vi "Spawn TCP Service.vi"(4 "Stop Module":refnum<user-event>, 6 "Message Queue":refnum<class "Delacor_lib_QMH_Message Queue.lvclass">, 7 "GenNet Protocol":refnum<class "GenNet Protocol.lvclass">, 8 "error in":errorcluster, 9 "Module ID":i32=-1, 11 "Connection ID":refnum<k5>) -> (0 "error out":errorcluster)   [LabVIEW 2022 SP3, in "GenNet-Server.lvlib"]
doc: "Spawns a new TCP/IP service for a networked client. Sets <b>Connection ID</b> reference, <b>Module ID</b>, <b>Caller MsqQ</b> queue reference and <b>Stop Module</b> event reference before running the service VI.\n\n____\nHAMPEL SOFTWARE ENGINEERING v3.8.0 (2023-12-18 14:41)"
uses:
  GenNet-Server.lvlib
  <vilib>/Delacor/Delacor QMH/Libraries/Message Queue_class/Delacor_lib_QMH_Message Queue.lvclass
  Stop Argument--cluster.ctl
  GenNet Protocols/GenNet Protocol.lvclass
  TCP Service.vi
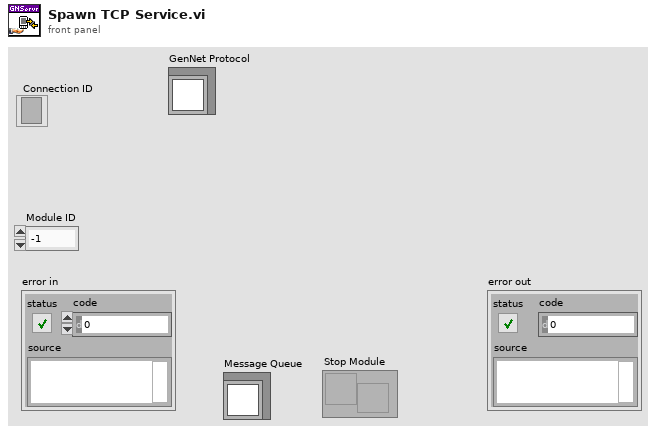
[diagram p1: front panel]
types:
  T1 = enum32{"Invalid", "Standard", "Closed", "Hidden", "Minimized", "Maximized"}
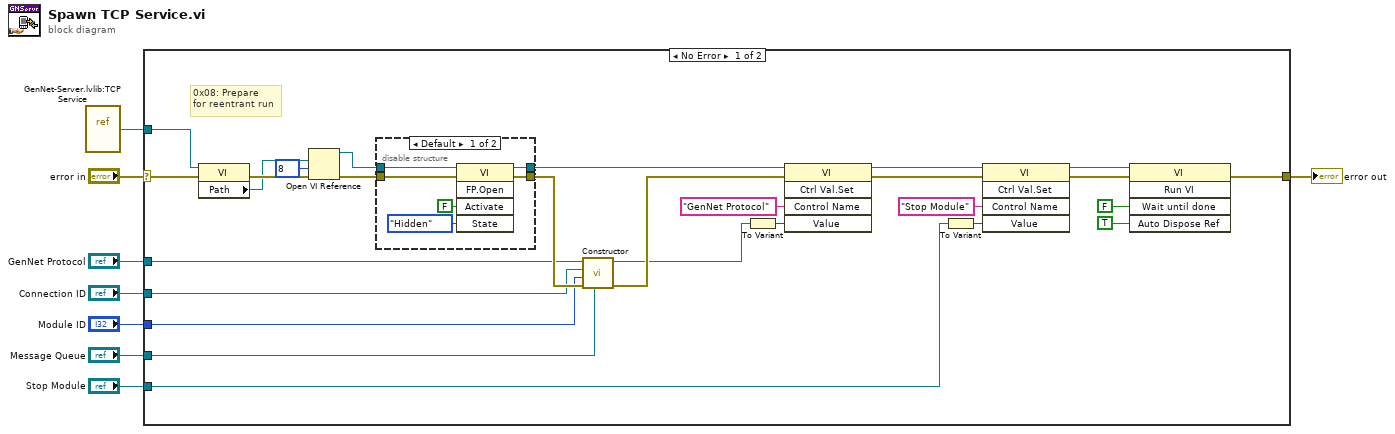
[diagram p0: block diagram]
diagram:
  n1 = vi-ref "GenNet-Server.lvlib:TCP Service.vi"() -> (w5:refnum<vi>)
  n2 = case shown="No Error" "error in" {
    selector: "error in" -> [w18 w44]
    tunnel: [w23 w44] -> w8
    tunnel: "Message Queue" -> [w13 _]
    tunnel: "Module ID" -> [w14 _]
    tunnel: w5 -> [w22 _]
    tunnel: "Connection ID" -> [w15 _]
    tunnel: "Stop Module" -> [w19 _]
    tunnel: "GenNet Protocol" -> [w17 _]
    frame No Error {
      # "0x08: Prepare \nfor reentrant run"
      n3 = property class="VI"(reference=w22, error in=w18) -> (error out=w26:errorcluster, "Path"=w25:path)  [unwired: 1 out]
      n4 = Open VI Reference(vi path=w25, options=8, error in (no error)=w26) -> (vi reference=w28:refnum<vi>, error out=w29:errorcluster)  [unwired: 3 in]
      n5 = disable-structure shown="Default" {
        disable-tunnel: [w41 w43] -> w24
        disable-tunnel: w29 -> [w40 w42]
        disable-tunnel: [w39 w42] -> w34
        disable-tunnel: w28 -> [w38 w43]
        frame condition #0 (active) {
          n6 = invoke class="VI" method="FP.Open"(reference=w38, error in=w40, "Activate"=FALSE ("Activate?"), "State"=T1."Hidden") -> (reference out=w41:refnum<vi>, error out=w39:errorcluster)  [unwired: 1 in, 3 out]
        }
        frame condition #1 {
        }
      }
      n7 = call-dynamic "Constructor.vi"("Message Queue"=w13, "error in (no error)"=w34, "Module ID"=w14, "Connection ID"=w15, "GenNet Protocol in"=w17) -> ("error out"=w35:errorcluster, "GenNet Protocol out"=w16:refnum<class "GenNet Protocol.lvclass">)  [unwired: 5 in]
      n8 = To Variant(anything=w16) -> (Variant=w30:variant)
      n9 = invoke class="VI" method="Ctrl Val.Set"(reference=w24, error in=w35, "Control Name"="GenNet Protocol", "Value"=w30) -> (reference out=w12:refnum<vi>, error out=w9:errorcluster)  [unwired: 1 in, 3 out]
      n10 = To Variant(anything=w19) -> (Variant=w21:variant)
      n11 = invoke class="VI" method="Ctrl Val.Set"(reference=w12, error in=w9, "Control Name"="Stop Module", "Value"=w21) -> (reference out=w11:refnum<vi>, error out=w10:errorcluster)  [unwired: 1 in, 3 out]
      n12 = invoke class="VI" method="Run VI"(reference=w11, error in=w10, "Wait until done"=FALSE ("Wait Until Done"), "Auto Dispose Ref"=TRUE ("Auto Dispose Reference")) -> (error out=w23:errorcluster)  [unwired: 1 in, 4 out]
    }
    frame Error {
    }
  }
  "error out" <- w8
